vi "Choosepicture.vi"(1 "Path":path) -> (7 "image data":T1, 8 "path":path)   [LabVIEW 2014]
uses:
  <vilib>/picture/picture.llb/imagedata.ctl
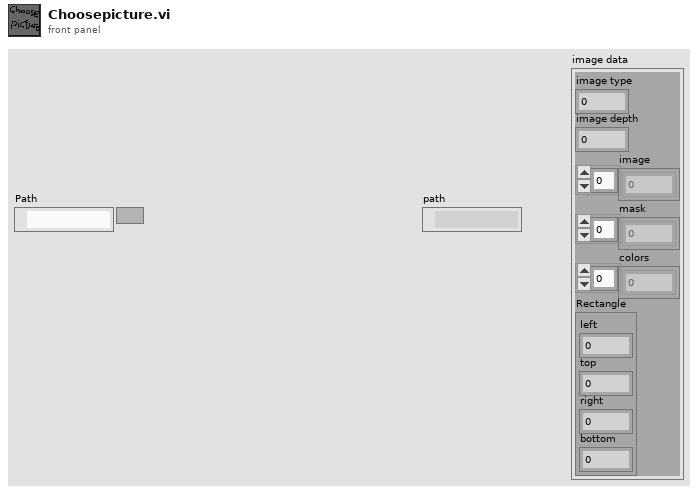
[diagram p1: front panel]
types:
  T1 = typedef "imagedata.ctl" = cluster{"image type":i32, "image depth":i32, "image":u8[], "mask":u8[], "colors":u32[], "Rectangle":cluster{"left":i16, "top":i16, "right":i16, "bottom":i16}}
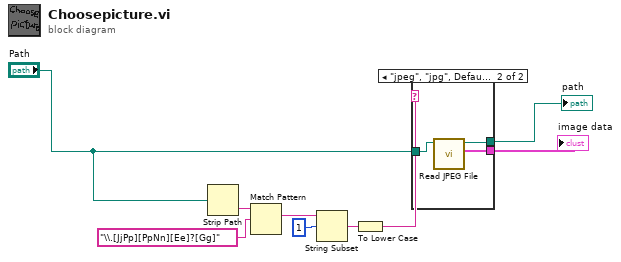
[diagram p0: block diagram]
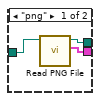
[diagram p2: hidden frame]
diagram:
  n1 = Strip Path(path="Path") -> (name=w3:string)  [unwired: 1 out]
  n2 = Match Pattern(string=w3, regular expression="\\.[JjPp][PpNn][Ee]?[Gg]") -> (match substring=w5:string)  [unwired: 1 in, 3 out]
  n3 = String Subset(string=w5, offset (0)=1) -> (substring=w7:string)  [unwired: 1 in]
  n4 = To Lower Case(string=w7) -> (all lower case string=w2:string)
  n5 = case shown="\"jpeg\", \"jpg\", Default" w2 {
    tunnel: "Path" -> [w12 w15]
    tunnel: [w11 w14] -> w8
    tunnel: [w10 w13] -> w9
    frame "png" {
      n6 = call <vilib>:"Read PNG File.vi"("path to PNG file"=w12) -> ("image data"=w10:T1, "path"=w11:path)  [unwired: 8 in, 1 out]
    }
    frame "jpeg", "jpg", Default {
      n7 = call <vilib>:"Read JPEG File.vi"("path to JPEG file"=w15) -> ("image data"=w13:T1, "path"=w14:path)  [unwired: 8 in, 1 out]
    }
  }
  "image data" <- w9
  "path" <- w8
